vi "Log position.vi"(8 "error in (no error)":errorcluster, 11 "ConfocalStage in":refnum<class "ConfocalStage.lvclass">) -> (0 "error out":errorcluster, 3 "ConfocalStage out":refnum<class "ConfocalStage.lvclass">)   [LabVIEW 2012, in "ConfocalStage.lvclass"]
uses:
  ConfocalStage.lvclass
  ConfocalStage.lvclass/ConfocalStage.ctl
  <vilib>/Utility/file.llb/Write To Spreadsheet File (string).vi
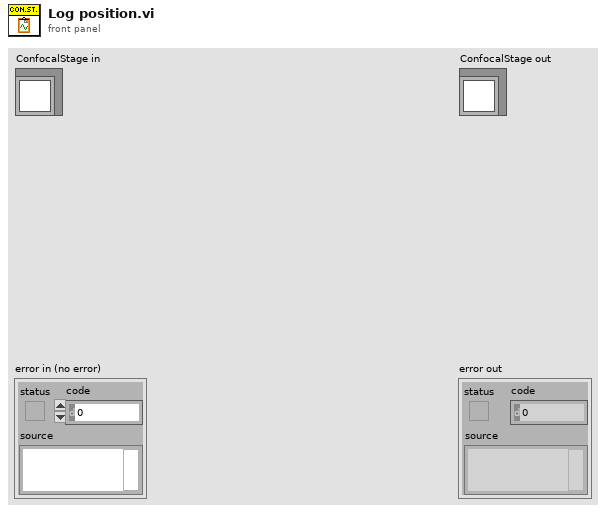
[diagram p1: front panel]
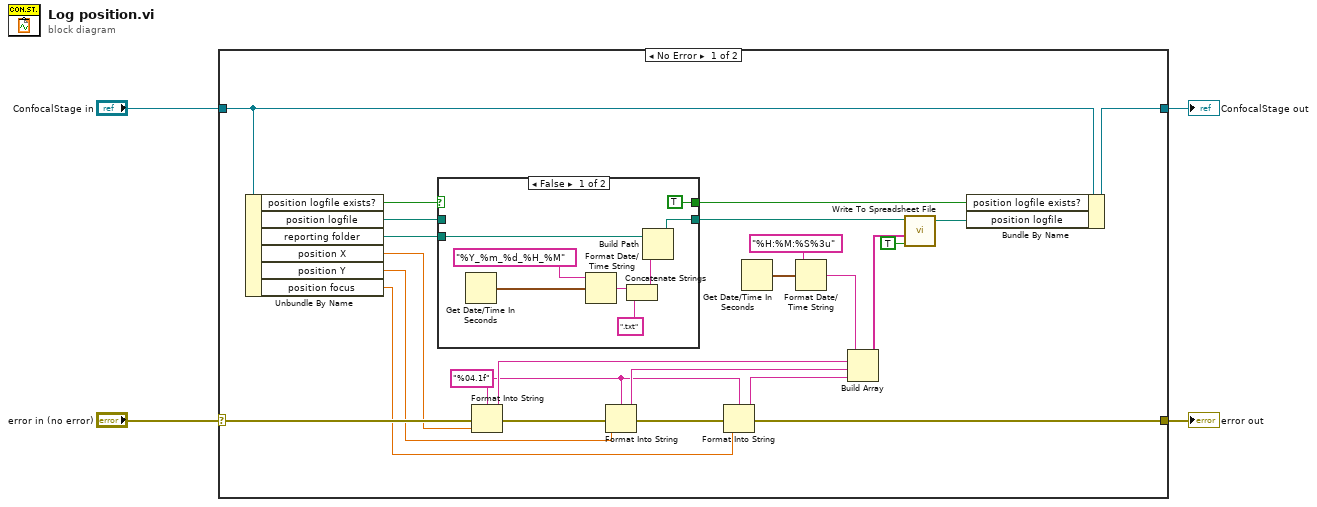
[diagram p0: block diagram]
diagram:
  n1 = case shown="No Error" "error in (no error)" {
    selector: "error in (no error)" -> [w19 w40]
    tunnel: [w14 w40] -> w3
    tunnel: [w8 w39] -> w1
    tunnel: "ConfocalStage in" -> [w9 w39]
    frame No Error {
      w5 = "%04.1f" ("format string")
      n2 = Unbundle By Name(w9) -> ("position logfile exists?"=w26:bool, "position logfile"=w27:path, "reporting folder"=w28:path, "position X"=w17:dbl, "position Y"=w13:dbl, "position focus"=w12:dbl)
      n3 = case shown="False" w26 {
        selector: w26 -> [_ w37]
        tunnel: w27 -> [_ w38]
        tunnel: [w34 w38] -> w18
        tunnel: w28 -> [w36 _]
        tunnel: [TRUE w37] -> w7
        frame False {
          n4 = Get Date/Time In Seconds() -> (seconds since 1Jan1904=w31:timestamp)
          n5 = Format Date/Time String(time format string (%c)="%Y_%m_%d_%H_%M", seconds (now)=w31) -> (date/time string=w32:string)  [unwired: 1 in]
          n6 = Concatenate Strings(w32, ".txt" ("string")) -> (w35:string)
          n7 = Build Path(base path=w36, name or relative path=w35) -> (appended path=w34:path)
        }
        frame True {
        }
      }
      n8 = Format Into String(format string=w5, error in=w19, w17) -> (resulting string=w25:string, error out=w16:errorcluster)  [unwired: 1 in]
      n9 = Format Into String(format string=w5, error in=w16, w13) -> (resulting string=w11:string, error out=w15:errorcluster)  [unwired: 1 in]
      n10 = Format Into String(format string=w5, error in=w15, w12) -> (resulting string=w10:string, error out=w14:errorcluster)  [unwired: 1 in]
      n11 = Get Date/Time In Seconds() -> (seconds since 1Jan1904=w22:timestamp)
      n12 = Format Date/Time String(time format string (%c)="%H:%M:%S%3u", seconds (now)=w22) -> (date/time string=w21:string)  [unwired: 1 in]
      n13 = Build Array(w21, w25, w11, w10) -> (w24:string[])
      n14 = call-poly <vilib>:"Write To Spreadsheet File.vi"("append to file? (new file:F)"=TRUE, "1D data"=w24, "file path (dialog if empty)"=w18) -> ("new file path (Not A Path if cancelled)"=w6:path)  [unwired: 5 in]
      n15 = Bundle By Name(cluster=w9, "position logfile exists?"=w7, "position logfile"=w6) -> (w8:refnum<class "ConfocalStage.lvclass">)
    }
    frame Error {
    }
  }
  "error out" <- w3
  "ConfocalStage out" <- w1
